vi "rotated_picture_init.vi"(11 "Picture FIle Name":string) -> (0 "appended path":path, 1 "Height":i16, 2 "Width":i16, 3 "RotatedPictureInfo":T1)   [LabVIEW 2020]
doc: "Initialize a PNG image to be rotated."
uses:
  Rotated_Picture_TypeDef.ctl
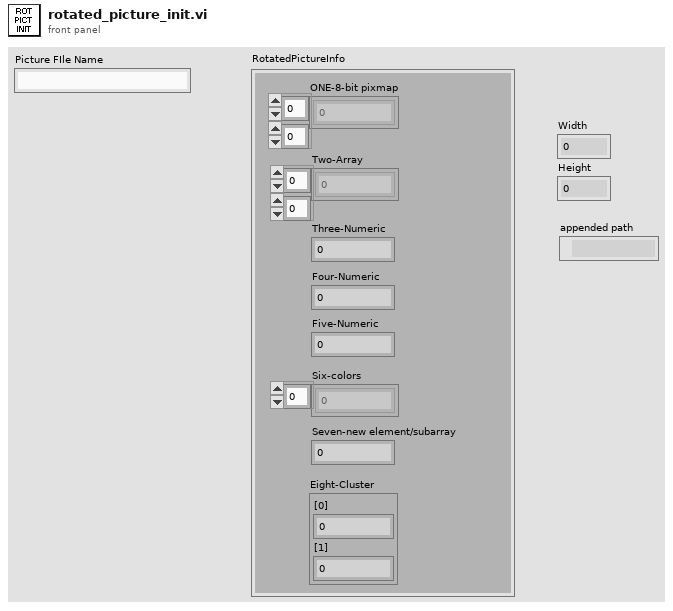
[diagram p1: front panel]
types:
  T1 = typedef "Rotated_Picture_TypeDef.ctl" = cluster{"ONE-8-bit pixmap":u8[][], "Two-Array":cdb[][], "Three-Numeric":i32, "Four-Numeric":i32, "Five-Numeric":cdb, "Six-colors":u32[], "Seven-new element/subarray":u32, "Eight-Cluster":cluster{"[0]":i32, "[1]":i32}}
  T2 = typedef "imagedata.ctl" = cluster{"image type":i32, "image depth":i32, "image":u8[], "mask":u8[], "colors":u32[], "Rectangle":cluster{"left":i16, "top":i16, "right":i16, "bottom":i16}}
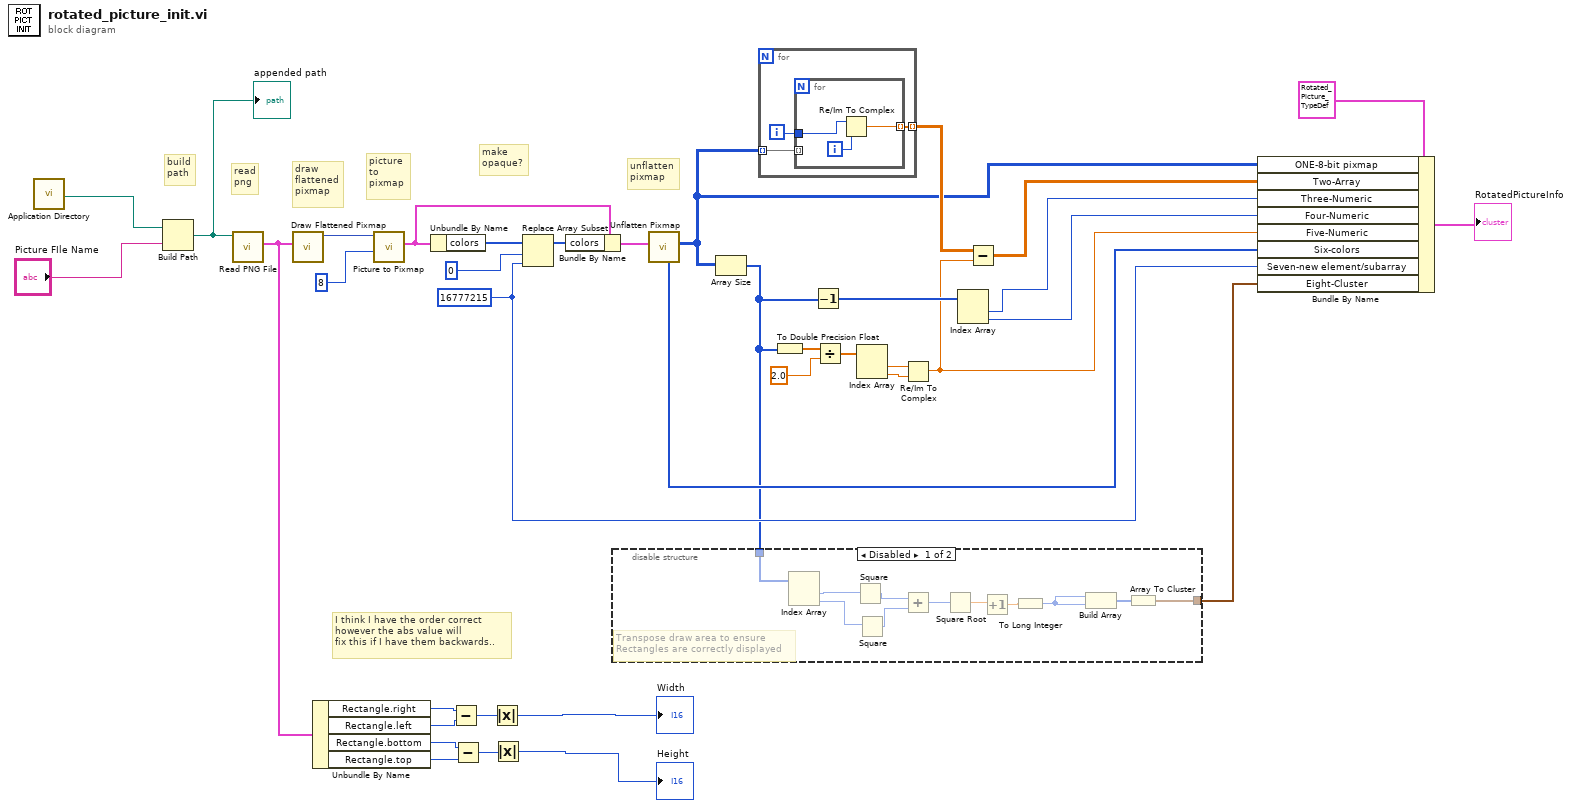
[diagram p0: block diagram]
diagram:
  w15 = u32 16777215 ("new element/subarray")
  # "I think I have the order correct\nhowever the abs value will\nfix this if I have them backwards.."
  # "unflatten\npixmap"
  # "make\nopaque?"
  # "picture\nto\npixmap"
  # "draw\nflattened\npixmap"
  # "read\npng"
  # "build\npath"
  n1 = call <vilib>:"Application Directory.vi"() -> ("Application Directory"=w12:path)
  n2 = Build Path(base path=w12, name or relative path="Picture FIle Name") -> (appended path=w29:path)
  "appended path" <- w29
  n3 = call <vilib>:"Read PNG File.vi"("path to PNG file"=w29) -> ("image data"=w9:T2)  [unwired: 8 in, 2 out]
  n4 = call <vilib>:"Draw Flattened Pixmap.vi"("image data"=w9) -> ("new picture"=w34:picture)  [unwired: 8 in]
  n5 = Unbundle By Name(w9) -> ("Rectangle.right"=w8:i16, "Rectangle.left"=w7:i16, "Rectangle.bottom"=w6:i16, "Rectangle.top"=w5:i16)
  n6 = call <vilib>:"Picture to Pixmap.vi"("depth"=8, "picture"=w34) -> ("image data"=w36:T2)  [unwired: 8 in, 1 out]
  n7 = Unbundle By Name(w36) -> ("colors"=w31:u32[])
  n8 = Subtract(x=w8, y=w7) -> (x-y=w4:i16)
  n9 = Subtract(x=w6, y=w5) -> (x-y=w3:i16)
  n10 = Absolute Value(x=w4) -> (abs(x)=→"Width":i16)
  n11 = Absolute Value(x=w3) -> (abs(x)=→"Height":i16)
  n12 = Replace Array Subset(array=w31, new element=w15, index=0) -> (w33:u32[])
  n13 = Bundle By Name(cluster=w36, "colors"=w33) -> (w37:T2)
  n14 = call <vilib>:"Unflatten Pixmap.vi"("image data"=w37) -> ("8-bit pixmap"=w21:u8[][], "colors"=w16:u32[])  [unwired: 4 in, 5 out]
  n15 = Array Size(array=w21) -> (size(s)=w11:i32[])
  n16 = disable-structure shown="Disabled" {
    disable-tunnel: w11 -> [w48 _]
    disable-tunnel: [w38 _] -> w14
    frame Disabled {
      # "Transpose draw area to ensure \nRectangles are correctly displayed"
      n17 = Index Array(array=w48) -> (element #1=w47:i32, element #2=w46:i32)  [unwired: 2 in]
      n18 = Square(x=w47) -> (x^2=w45:i32)
      n19 = Square(x=w46) -> (x^2=w44:i32)
      n20 = Add(x=w45, y=w44) -> (x+y=w43:i32)
      n21 = Square Root(x=w43) -> (sqrt(x)=w42:dbl)
      n22 = Increment(x=w42) -> (x+1=w41:dbl)
      n23 = To Long Integer(number=w41) -> (32bit integer=w40:i32)
      n24 = Build Array(w40, w40) -> (w39:i32[])
      n25 = Array To Cluster(array=w39) -> (cluster=w38:cluster{"[0]":i32, "[1]":i32})
    }
    frame Enabled {
    }
  }
  n26 = for {
    tunnel: [w50] -> w23 mode=indexing
    tunnel: w21 -> [w49] mode=indexing
    i -> [w51]
    n27 = for {
      tunnel: w51 -> [w54]
      tunnel: [w53] -> w50 mode=indexing
      tunnel: w49 -> [_] mode=indexing
      i -> [w52]
      n28 = Re/Im To Complex(1:w52, 2:w54) -> (0:w53:cdb)
    }
  }
  n29 = To Double Precision Float(number=w11) -> (double precision float=w10:dbl[])
  n30 = Decrement(x=w11) -> (x-1=w28:i32[])
  n31 = Divide(x=w10, y=2.0) -> (x/y=w25:dbl[])
  n32 = Index Array(array=w25) -> (element #1=w26:dbl, element #2=w27:dbl)  [unwired: 2 in]
  n33 = Re/Im To Complex(1:w27, 2:w26) -> (0:w17:cdb)
  n34 = Index Array(array=w28) -> (element #1=w19:i32, element #2=w18:i32)  [unwired: 2 in]
  n35 = Subtract(x=w23, y=w17) -> (x-y=w20:cdb[][])
  n36 = Bundle By Name(cluster=T1 {"ONE-8-bit pixmap"=[], "Two-Array"=[], "Three-Numeric"=0, "Four-Numeric"=0, "Five-Numeric"=0.0+0.0i, "Six-colors"=[], "Seven-new element/subarray"=0, "Eight-Cluster"={"[0]"=0, "[1]"=0}} ("RotatedPictureInfo"), "ONE-8-bit pixmap"=w21, "Two-Array"=w20, "Three-Numeric"=w19, "Four-Numeric"=w18, "Five-Numeric"=w17, "Six-colors"=w16, "Seven-new element/subarray"=w15, "Eight-Cluster"=w14) -> (→"RotatedPictureInfo":T1)
